vi "Marshal.vi"(8 "error in (no error)":errorcluster, 11 "int32 in":refnum<class "uint32.lvclass">) -> (0 "error out":errorcluster, 2 "Buffer":u8[](array[numeric]), 3 "int32 out":refnum<class "uint32.lvclass">)   [LabVIEW 2020, in "Protobuf RAW.lvlib" / "uint32.lvclass"]
uses:
  uint32.lvclass
  uint32.lvclass/uint32.ctl
  9300a24b-3453-4a93-b2ba-fd010a7e1bbf.vi
  9300a24b-3453-4a93-b2ba-fd010a7e1bbf.vi/0f065a35-b637-42bd-ae45-04c3465bdb97.vi
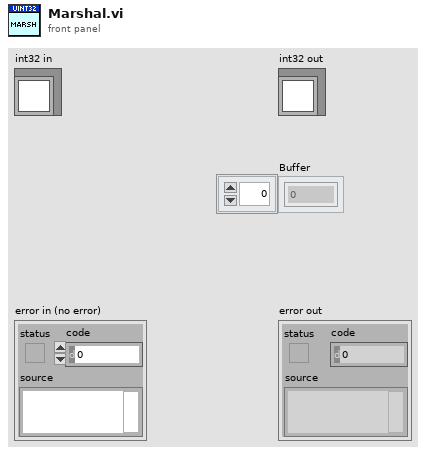
[diagram p1: front panel]
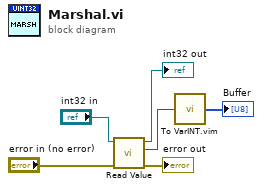
[diagram p0: block diagram]
diagram:
  n1 = call "Read Value.vi"("error in (no error)"="error in (no error)", "int32 in"="int32 in") -> ("error out"=→"error out":errorcluster, "Value"=w1:u32, "int32 out"=→"int32 out":refnum<class "uint32.lvclass">)  [unwired: 7 in]
  n2 = call "To VarINT.vim"("Integer"=w1) -> ("LEB128"=→"Buffer":u8[])
